vi "loadLutFile.vi"(8 "error in":errorcluster, 9 "Path to LUT file":path, 10 "axis":i32, 11 "connection ID":refnum<k5>) -> (0 "error out":errorcluster, 2 "axis_out":i32, 3 "connection ID 2":refnum<k5>)   [LabVIEW 2016, in "AMC_VIs.lvlib"]
doc: "This VI loads the LUT-file pointed to by 'path to LUT file' into the device for the specified axis"
uses:
  AMC_VIs.lvlib
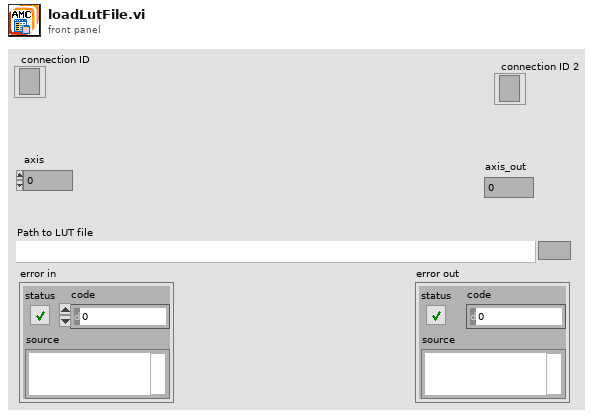
[diagram p1: front panel]
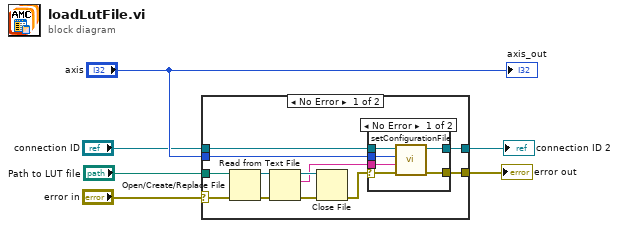
[diagram p0: block diagram]
diagram:
  n1 = case shown="No Error" "error in" {
    selector: "error in" -> [w9 w28]
    tunnel: [w10 w28] -> w1
    tunnel: [w17 w27] -> w2
    tunnel: "connection ID" -> [w18 w27]
    tunnel: "axis" -> [w12 _]
    tunnel: "Path to LUT file" -> [w8 _]
    frame No Error {
      n2 = Open/Create/Replace File(file path (use dialog)=w8, error in=w9) -> (refnum out=w7:refnum<file>, error out=w16:errorcluster)  [unwired: 4 in, 1 out]
      n3 = Read from Text File(file (use dialog)=w7, error in=w16) -> (refnum out=w14:refnum<file>, text=w13:string, error out=w15:errorcluster)  [unwired: 2 in, 1 out]
      n4 = Close File(refnum=w14, error in=w15) -> (error out=w11:errorcluster)  [unwired: 1 out]
      n5 = case shown="No Error" w11 {
        selector: w11 -> [w22 w26]
        tunnel: w18 -> [w24 w25]
        tunnel: [w20 w25] -> w17
        tunnel: w13 -> [w19 _]
        tunnel: w12 -> [w23 _]
        tunnel: [w21 w26] -> w10
        frame No Error {
          n6 = call "setConfigurationFile.vi"("error in"=w22, "content"=w19, "axis"=w23, "connection ID"=w24) -> ("error out"=w21:errorcluster, "connection ID"=w20:refnum<k5>)  [unwired: 5 in, 1 out]
        }
        frame Error {
        }
      }
    }
    frame Error {
    }
  }
  "error out" <- w1
  "connection ID 2" <- w2
  "axis_out" <- "axis"
